vi "Transfer Display Data (SubVI).vi"(5 "Tranfer Time":u32=50000, 7 "EOF?":bool, 11 "Read":bool) -> (0 "Data Valid":bool, 3 "Data Out":u64)   [LabVIEW 2015]
uses:
  Controls (FPGA)/Send Display Data.ctl
  <vilib>/rvi/Emulation/niFpgaEmulationIsFPGAContextNoSignature.vi
  <vilib>/rvi/Emulation/niFpgaSctlEmulationGetInTimedLoop.vi
  <vilib>/rvi/errors/niFpgaSetErrorForExecOnDevCompSimple.vi
  <vilib>/rvi/eio/common/nirviEmuReportErrorAndStop.vi
  <vilib>/rvi/DataTransferAndStorage/Container/Common/niFpgaContainerGetUniqueNameForEmu.vi
  <vilib>/rvi/FIFO/Fifo_Resource/nirvififoEmulationSetSize.vi
  <vilib>/rvi/FIFO/Fifo_Resource/nirviFifoEmulationQueueMgr.vi
  <instcachedir>/0/nirviFifoEmulationQueueMgr_E5CAEC123FF24DC58D834DCA3CDAA9B5.lvgen/nirviFifoEmulationQueueMgr_E5CAEC123FF24DC58D834DCA3CDAA9B5_006.vi
  <vilib>/Utility/error.llb/Clear Errors.vi
  <vilib>/rvi/FIFO/Fifo_Resource/nirvififoEmulationCreateLock.vi
  <vilib>/rvi/Emulation/niFpgaProcessEmulError.vi
  <vilib>/rvi/FIFO/Fifo_Resource/nirvififoEmulationObtainLock.vi
  <vilib>/rvi/FIFO/Fifo_Resource/nirvififoEmulationReleaseLock.vi
  <vilib>/rvi/occurrence/nirviWaitOnOccurrenceBase.vi
  <vilib>/rvi/errors/nirviReportUnexpectedCaseInternalError.vi
  <vilib>/rvi/errors/nirviReportUnexpectedCaseInternalError (U32).vi
  <vilib>/rvi/DataTransferAndStorage/Container/XNode/niFpgaContainer.xnode
  <vilib>/rvi/FIFO/Fifo_Resource/nirvififoEmulationRead.vi
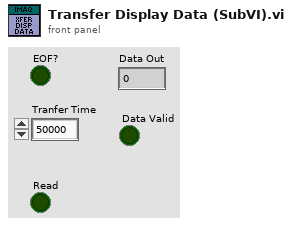
[diagram p1: front panel]
types:
  T1 = typedef "Send Display Data.ctl" = enum16{"Wait", "Pass N Clock Cycles", "Send Data Lower 64", "Send Data Upper 64"}
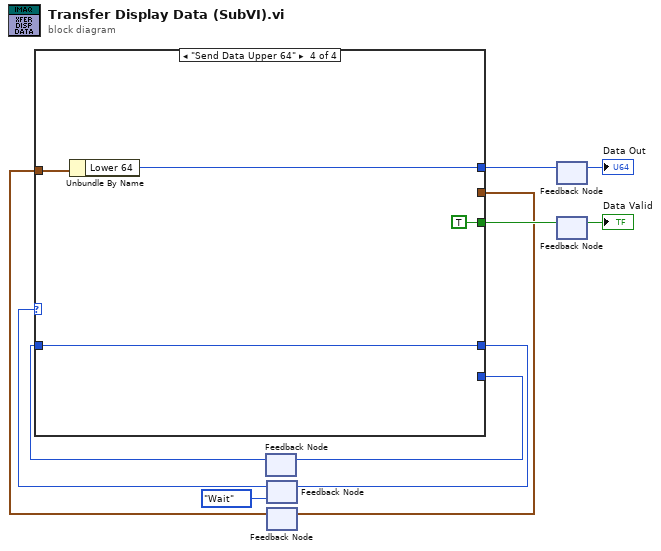
[diagram p0: block diagram]
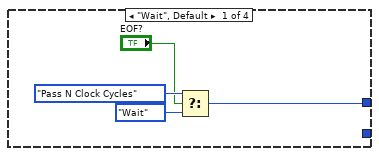
[diagram p2: hidden frame]
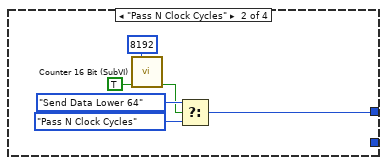
[diagram p3: hidden frame]
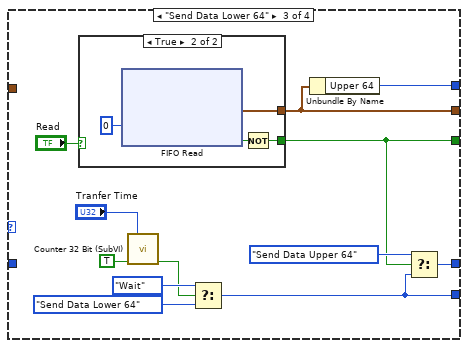
[diagram p4: hidden frame]
diagram:
  n1 = feedback #1() -> (w9:T1)  [unwired: 1 in]
  n2 = feedback #2(Send_Display_Data."Wait" ("f")) -> (w4:T1)
  n3 = feedback #3() -> (w7:cluster{"Lower 64":u64, "Upper 64":u64})  [unwired: 1 in]
  n4 = case shown="\"Send Data Upper 64\"" w4 {
    tunnel: [w13 w19 w32 w39] -> w3
    tunnel: [_ _ w30 _] -> w6
    tunnel: [_ _ w31 TRUE] -> w11
    tunnel: w7 -> [_ _ _ w41]
    tunnel: [_ _ w29 w40] -> w10
    tunnel: [_ _ w23 _] -> w8
    tunnel: w9 -> [_ _ _ w39]
    frame "Wait", Default {
      n5 = Select(t=Send_Display_Data."Pass N Clock Cycles" ("f"), s="EOF?", f=Send_Display_Data."Wait") -> (s? t:f=w13:T1)
    }
    frame "Pass N Clock Cycles" {
      n6 = call "Counter 16 Bit (SubVI).vi"("Max. Count"=u16 8192, "Enable"=TRUE) -> ("Count End?"=w16:bool)  [unwired: 11 in, 2 out]
      n7 = Select(t=Send_Display_Data."Send Data Lower 64" ("f"), s=w16, f=Send_Display_Data."Pass N Clock Cycles") -> (s? t:f=w19:T1)
    }
    frame "Send Data Lower 64" {
      n8 = case shown="True" "Read" {
        tunnel: [_ w35] -> w31
        tunnel: [_ w34] -> w30
        frame False {
        }
        frame True {
          n9 = xnode ("FIFO Read")("Timeout"=0) -> ("Element"=w34:cluster{"Lower 64":u64, "Upper 64":u64}, "Timed Out?"=w36:bool)  [unwired: 1 in, 1 out]
          n10 = Not(x=w36) -> (.not. x?=w35:bool)
        }
      }
      n11 = call "Counter 32 Bit (SubVI).vi"("Max. Count"="Tranfer Time", "Enable"=TRUE) -> ("Count End?"=w24:bool)  [unwired: 11 in, 2 out]
      n12 = Select(t=Send_Display_Data."Wait" ("f"), s=w24, f=Send_Display_Data."Send Data Lower 64") -> (s? t:f=w23:T1)
      n13 = Unbundle By Name(w30) -> ("Upper 64"=w29:u64)
      n14 = Select(t=Send_Display_Data."Send Data Upper 64" ("f"), s=w31, f=w23) -> (s? t:f=w32:T1)
    }
    frame "Send Data Upper 64" {
      n15 = Unbundle By Name(w41) -> ("Lower 64"=w40:u64)
    }
  }
  n16 = feedback-in #1(w8) -> ()
  n17 = feedback-in #2(w3) -> ()
  n18 = feedback-in #3(w6) -> ()
  n19 = feedback-in #4(w10) -> ()
  n20 = feedback #4() -> (→"Data Out":u64)  [unwired: 1 in]
  n21 = feedback-in #5(w11) -> ()
  n22 = feedback #5() -> (→"Data Valid":bool)  [unwired: 1 in]
